vi "ScpiSendReplyLog.vi"(6 "TCP Timeout mS":i32=15000, 7 "error in (no error)":errorcluster, 8 "Command":string, 9 "TCP port":u16=5025 min=1025 step=1, 10 "IP Address":string="localhost") -> (0 "Error out":errorcluster, 3 "Reply":string)   [LabVIEW 2009]
doc: "Sends a SCPI command to an instrument.\nWaits for the reply.\nReply string must end in NewLine character."
panel:
  out "size (in bytes)":i64
  out "error out":errorcluster
  in  "Instrument":T1(ring)
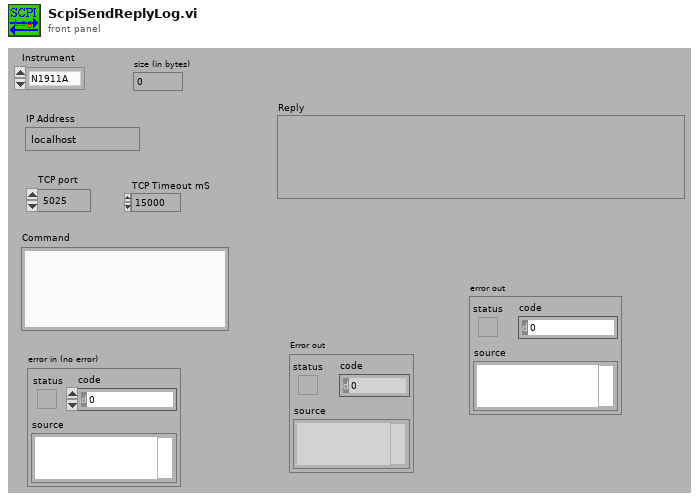
[diagram p1: front panel]
types:
  T1 = enum16{"N1911A", "Siggen", "34980a", "E4418B", "Rvp8"}
  T2 = enum16{"Read_SCPI_Log_Status", "No_SCPI_Log", "Log_SCPI", "Reset"}
  T3 = enum16{"open", "replace", "create", "open or create", "replace or create", "replace or create with confirmation"}
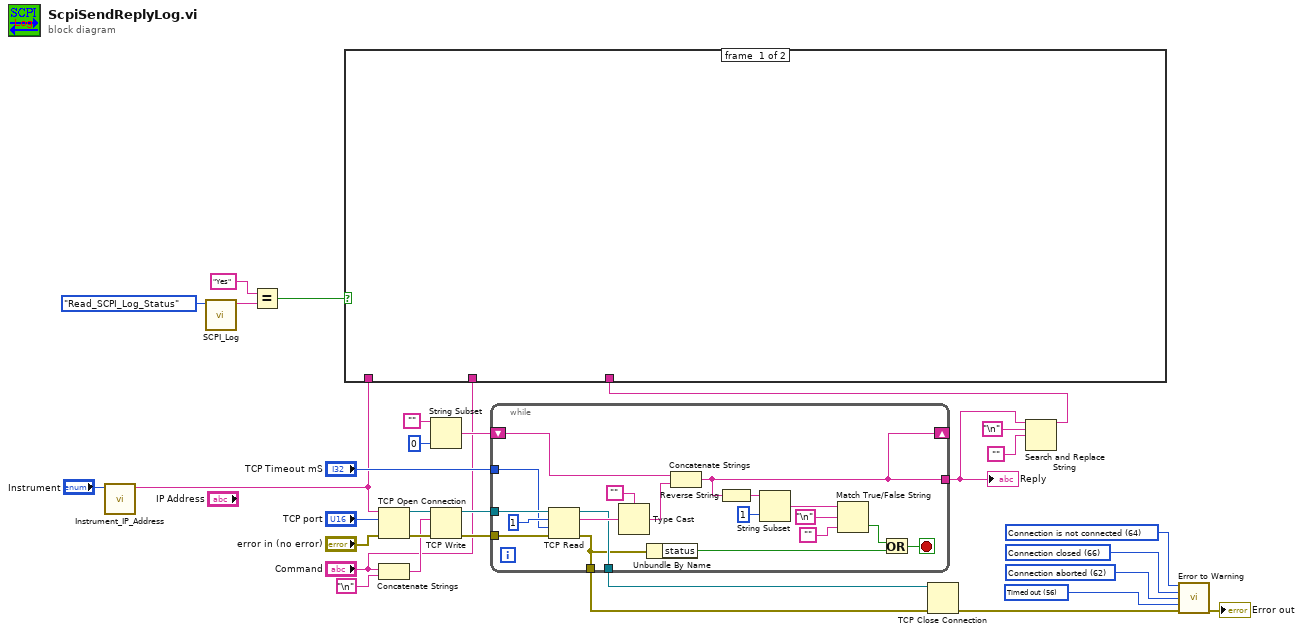
[diagram p0: block diagram]
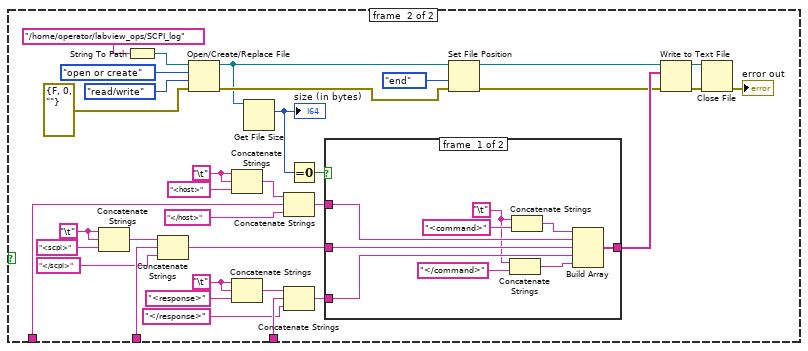
[diagram p2: hidden frame]
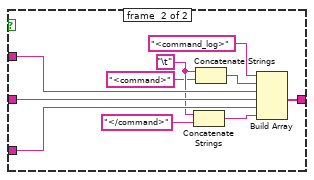
[diagram p3: hidden frame]
diagram:
  w15 = 56 items=["No Error", "Argument Error", "Memory Full", "Out of Zone", "End of File", "File Already Open", "Generic File IO Error", "File Not Found", "File Permission Error", "Disk Full", "Duplicate Path", "Too Many Files Open", "Not Enabled", "Resource File Not Found", "Cannot Add Resource", "Resource Not Found", "Image Not Found", "Image Memory Error", "Pen Does Not Exist", "Config Bad Type", "Config Token Not Found", "Config Parse Error", "Config Memory Error", "Bad External Code Format", "Bad External Code Offset", "External Code Not Present", "Null Window", "Destroy Window Mixup", "Null Menu", "Print Aborted", "Bad Print Record", "Print Driver Error", "Windows Error During Print", "Memory Error During Print", "Print Dialog Error", "Generic Print Error", "Invalid Device Refnum", "Device Not Found", "Device Parameter Error", "Device Unit Error", "Can't Open Device", "Device Call Aborted", "Generic Error", "Cancelled By User", "Object ID Too Low", "Object ID Too High", "Object Not In Heap", "Unknown Heap", "Bad DefProc ID", "DefProc Not In Table", "Message Out Of Range", "Null Method", "Unknown Message", "Manager Call Not Supported", "Bad address", "Connection In progress", "Timed out", "Connection is already in progress", "Network attribute not supported", "Network error", "Address in use", "System out of memory", "Connection aborted", "Connection refused", "Connection is not connected", "Connection is already connected", "Connection closed", "Initialize error (interapplication manager)", "Bad occurrence", "Wait on unbound occurrence handler", "Occurrence queue overflow", "Bad path", "Semaphore not signaled", "Unrecognized type (interapplication manager)"] ("1st Error to Convert")
  w26 = 62 items=["No Error", "Argument Error", "Memory Full", "Out of Zone", "End of File", "File Already Open", "Generic File IO Error", "File Not Found", "File Permission Error", "Disk Full", "Duplicate Path", "Too Many Files Open", "Not Enabled", "Resource File Not Found", "Cannot Add Resource", "Resource Not Found", "Image Not Found", "Image Memory Error", "Pen Does Not Exist", "Config Bad Type", "Config Token Not Found", "Config Parse Error", "Config Memory Error", "Bad External Code Format", "Bad External Code Offset", "External Code Not Present", "Null Window", "Destroy Window Mixup", "Null Menu", "Print Aborted", "Bad Print Record", "Print Driver Error", "Windows Error During Print", "Memory Error During Print", "Print Dialog Error", "Generic Print Error", "Invalid Device Refnum", "Device Not Found", "Device Parameter Error", "Device Unit Error", "Can't Open Device", "Device Call Aborted", "Generic Error", "Cancelled By User", "Object ID Too Low", "Object ID Too High", "Object Not In Heap", "Unknown Heap", "Bad DefProc ID", "DefProc Not In Table", "Message Out Of Range", "Null Method", "Unknown Message", "Manager Call Not Supported", "Bad address", "Connection In progress", "Connection timed out", "Connection is already in progress", "Network attribute not supported", "Network error", "Address in use", "System out of memory", "Connection aborted", "Connection refused", "Connection is not connected", "Connection is already connected", "Connection closed", "Initialize error (interapplication manager)", "Bad occurrence", "Wait on unbound occurrence handler", "Occurrence queue overflow", "Bad path", "Semaphore not signaled", "Unrecognized type (interapplication manager)"] ("1st Error to Convert")
  w27 = 66 items=["No Error", "Argument Error", "Memory Full", "Out of Zone", "End of File", "File Already Open", "Generic File IO Error", "File Not Found", "File Permission Error", "Disk Full", "Duplicate Path", "Too Many Files Open", "Not Enabled", "Resource File Not Found", "Cannot Add Resource", "Resource Not Found", "Image Not Found", "Image Memory Error", "Pen Does Not Exist", "Config Bad Type", "Config Token Not Found", "Config Parse Error", "Config Memory Error", "Bad External Code Format", "Bad External Code Offset", "External Code Not Present", "Null Window", "Destroy Window Mixup", "Null Menu", "Print Aborted", "Bad Print Record", "Print Driver Error", "Windows Error During Print", "Memory Error During Print", "Print Dialog Error", "Generic Print Error", "Invalid Device Refnum", "Device Not Found", "Device Parameter Error", "Device Unit Error", "Can't Open Device", "Device Call Aborted", "Generic Error", "Cancelled By User", "Object ID Too Low", "Object ID Too High", "Object Not In Heap", "Unknown Heap", "Bad DefProc ID", "DefProc Not In Table", "Message Out Of Range", "Null Method", "Unknown Message", "Manager Call Not Supported", "Bad address", "Connection In progress", "Connection timed out", "Connection is already in progress", "Network attribute not supported", "Network error", "Address in use", "System out of memory", "Connection aborted", "Connection refused", "Connection is not connected", "Connection is already connected", "Connection closed", "Initialize error (interapplication manager)", "Bad occurrence", "Wait on unbound occurrence handler", "Occurrence queue overflow", "Bad path", "Semaphore not signaled", "Unrecognized type (interapplication manager)"] ("1st Error to Convert")
  w28 = 64 items=["No Error", "Argument Error", "Memory Full", "Out of Zone", "End of File", "File Already Open", "Generic File IO Error", "File Not Found", "File Permission Error", "Disk Full", "Duplicate Path", "Too Many Files Open", "Not Enabled", "Resource File Not Found", "Cannot Add Resource", "Resource Not Found", "Image Not Found", "Image Memory Error", "Pen Does Not Exist", "Config Bad Type", "Config Token Not Found", "Config Parse Error", "Config Memory Error", "Bad External Code Format", "Bad External Code Offset", "External Code Not Present", "Null Window", "Destroy Window Mixup", "Null Menu", "Print Aborted", "Bad Print Record", "Print Driver Error", "Windows Error During Print", "Memory Error During Print", "Print Dialog Error", "Generic Print Error", "Invalid Device Refnum", "Device Not Found", "Device Parameter Error", "Device Unit Error", "Can't Open Device", "Device Call Aborted", "Generic Error", "Cancelled By User", "Object ID Too Low", "Object ID Too High", "Object Not In Heap", "Unknown Heap", "Bad DefProc ID", "DefProc Not In Table", "Message Out Of Range", "Null Method", "Unknown Message", "Manager Call Not Supported", "Bad address", "Connection In progress", "Connection timed out", "Connection is already in progress", "Network attribute not supported", "Network error", "Address in use", "System out of memory", "Connection aborted", "Connection refused", "Connection is not connected", "Connection is already connected", "Connection closed", "Initialize error (interapplication manager)", "Bad occurrence", "Wait on unbound occurrence handler", "Occurrence queue overflow", "Bad path", "Semaphore not signaled", "Unrecognized type (interapplication manager)"] ("1st Error to Convert")
  n1 = call "Instrument_IP_Address.vi"("Instrument"="Instrument") -> ("IP Address"=w9:string)  [unwired: 9 in, 1 out]
  n2 = call "SCPI_Log.vi"("SCOP Log In"=T2."Read_SCPI_Log_Status") -> ("SCPI Log Out"=w10:string)  [unwired: 10 in]
  n3 = Equal?(x="Yes" ("SCPI Log Out"), y=w10) -> (x = y?=w11:bool)
  n4 = TCP Open Connection(address=w9, remote port or service name="TCP port", error in (no error)="error in (no error)") -> (connection ID=w24:refnum<k5>, error out=w22:errorcluster)  [unwired: 2 in]
  n5 = Concatenate Strings("Command", "\n") -> (w7:string)
  n6 = String Subset(string="", length (rest)=0) -> (substring=w16:string)  [unwired: 1 in]
  n7 = TCP Write(connection ID=w24, data in=w7, error in (no error)=w22) -> (connection ID out=w23:refnum<k5>, error out=w21:errorcluster)  [unwired: 1 in, 1 out]
  n8 = while {
    tunnel: w23 -> [w49]
    tunnel: w21 -> [w48]
    shift-right: [w35] -> _
    shift-left: w16 -> [w44]
    tunnel: [w37] -> w20
    tunnel: [w43] -> w19
    tunnel: [w35] -> w4
    tunnel: "TCP Timeout mS" -> [w36]
    stop <- w32 stop-if-true
    n9 = TCP Read(connection ID=w49, bytes to read=1, error in (no error)=w48, 9:w36) -> (connection ID out=w43:refnum<k5>, data out=w47:string, error out=w37:errorcluster)  [unwired: 1 in]
    n10 = Type Cast(type="", x=w47) -> (*(type *) &x=w45:string)
    n11 = Unbundle By Name(w37) -> ("status"=w33:bool)
    n12 = Concatenate Strings(w44, w45) -> (w35:string)
    n13 = Reverse String(1:w35) -> (0:w42:string)
    n14 = String Subset(string=w42, length (rest)=1) -> (substring=w40:string)  [unwired: 1 in]
    n15 = Match True/False String(2:"", 3:"\n", 4:w40) -> (0:w34:bool)  [unwired: 1 out]
    n16 = Or(x=w34, y=w33) -> (x .or. y?=w32:bool)
  }
  "Reply" <- w4
  n17 = TCP Close Connection(connection ID=w19, error in (no error)=w20) -> (error out=w30:errorcluster)  [unwired: 1 in, 1 out]
  n18 = Search and Replace String(input string=w4, search string="\n", replace string="") -> (result string=w3:string)  [unwired: 5 in, 3 out]
  n19 = case shown="True" w11 {
    tunnel: w9 -> [_ w66]
    tunnel: "Command" -> [_ w73]
    tunnel: w3 -> [_ w70]
    frame #0 {
    }
    frame #1 {
      w61 = "\t"
      w56 = "\t"
      w54 = "\t"
      n20 = Concatenate Strings(w56, w56, "<scpi>") -> (w62:string)
      n21 = String To Path(string="/home/operator/labview_ops/SCPI_log" ("SCPI Log Out")) -> (path=w83:path)
      n22 = Concatenate Strings(w62, w73, "</scpi>") -> (w72:string)
      n23 = Open/Create/Replace File(file path (use dialog)=w83, error in=errorcluster {"status"=FALSE, "code"=0, "source"=""}, operation (0:open)=T3."open or create", access (0:read/write)=enum16{"read/write", "read-only", "write-only"}."read/write") -> (refnum out=w69:refnum<file>, error out=w77:errorcluster)  [unwired: 2 in, 1 out]
      n24 = Concatenate Strings(w54, w54, "<host>") -> (w64:string)
      n25 = Concatenate Strings(w61, w61, "<response>") -> (w59:string)
      n26 = Get File Size(file=w69) -> (size (in bytes)=w67:i64)  [unwired: 1 in, 2 out]
      "size (in bytes)" <- w67
      n27 = Concatenate Strings(w64, w66, "</host>") -> (w74:string)
      n28 = Concatenate Strings(w59, w70, "</response>") -> (w71:string)
      n29 = Equal To 0?(x=w67) -> (x = 0?=w68:bool)
      n30 = case shown="False" w68 {
        tunnel: w72 -> [w92 w103]
        tunnel: w71 -> [w91 w102]
        tunnel: [w90 w101] -> w80
        tunnel: w74 -> [w93 w100]
        frame #0 {
          w85 = "\t"
          n31 = Concatenate Strings(w85, "</command>") -> (w89:string)
          n32 = Concatenate Strings(w85, "<command>") -> (w86:string)
          n33 = Build Array(w86, w93, w92, w91, w89) -> (w90:string[])
        }
        frame #1 {
          w98 = "\t"
          n34 = Concatenate Strings(w98, "</command>") -> (w95:string)
          n35 = Concatenate Strings(w98, "<command>") -> (w94:string)
          n36 = Build Array("<command_log>", w94, w100, w103, w102, w95) -> (w101:string[])
        }
      }
      n37 = Set File Position(refnum=w69, from (0:start)=enum16{"start", "end", "current"}."end", error in=w77) -> (refnum out=w81:refnum<file>, error out=w76:errorcluster)  [unwired: 1 in]
      n38 = Write to Text File(file (use dialog)=w81, text=w80, error in=w76) -> (refnum out=w52:refnum<file>, error out=w51:errorcluster)  [unwired: 1 in, 1 out]
      n39 = Close File(refnum=w52, error in=w51) -> (error out=→"error out":errorcluster)  [unwired: 1 out]
    }
  }
  n40 = call <vilib>:"Error to Warning.vi"("1st Error to Convert"=w28, "2nd Error to Convert"=w27, "3rd Error to Convert"=w26, "4th Error to Convert"=w15, "error in"=w30) -> ("warning out"=→"Error out":errorcluster)  [unwired: 10 in]
